vi "add scan field(SubVI).vi"(10 "字符串":string) -> (0 "布尔 3":bool, 2 "连接的字符串":string)   [LabVIEW 2019, in "Add Seq.lvlib"]
uses:
  Add Seq.lvlib
  SubVI.lvlib
panel:
  in  "Number of Step":i32=2
  in  "Step Delay(secs)":dbl
  in  "Increments(Oe)":dbl=10.0
  in  "cancel":bool
  in  "ok":bool
  in  "Approach":i32(ring)=1 items=["Linear", "NoOvershoot", "Oscillate", "Sweep"]
  in  "End Mode":i32(ring) items=["Persistent", "Driven"]
  in  "Rate(Oe/secs)":dbl=100.0 min=0.0 max=100.0
  in  "Final Field(Oe)":dbl min=-140000.0 max=140000.0
  in  "Initial Field(Oe)":dbl min=-140000.0 max=140000.0
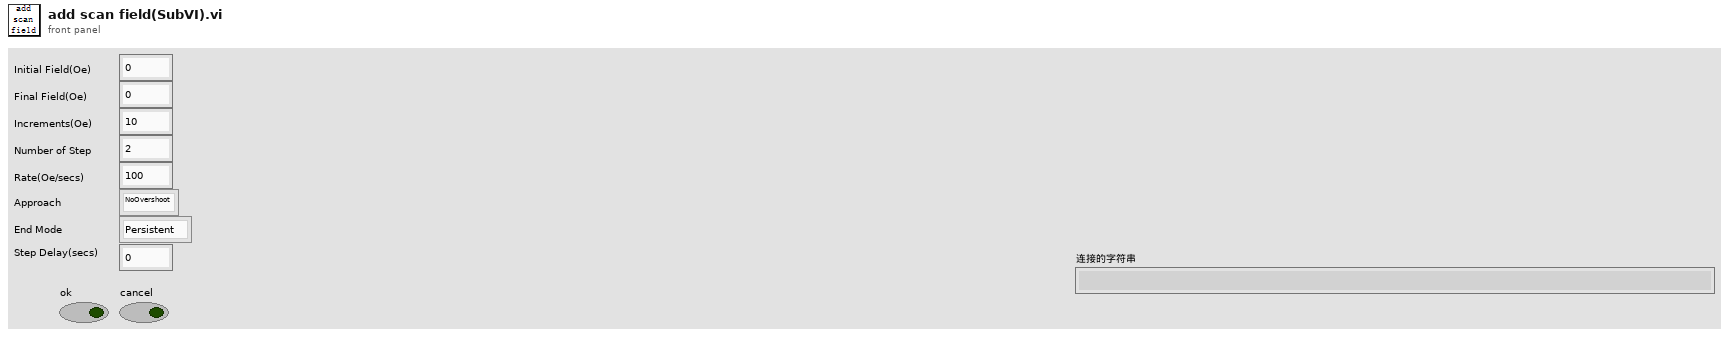
[diagram p1: front panel]
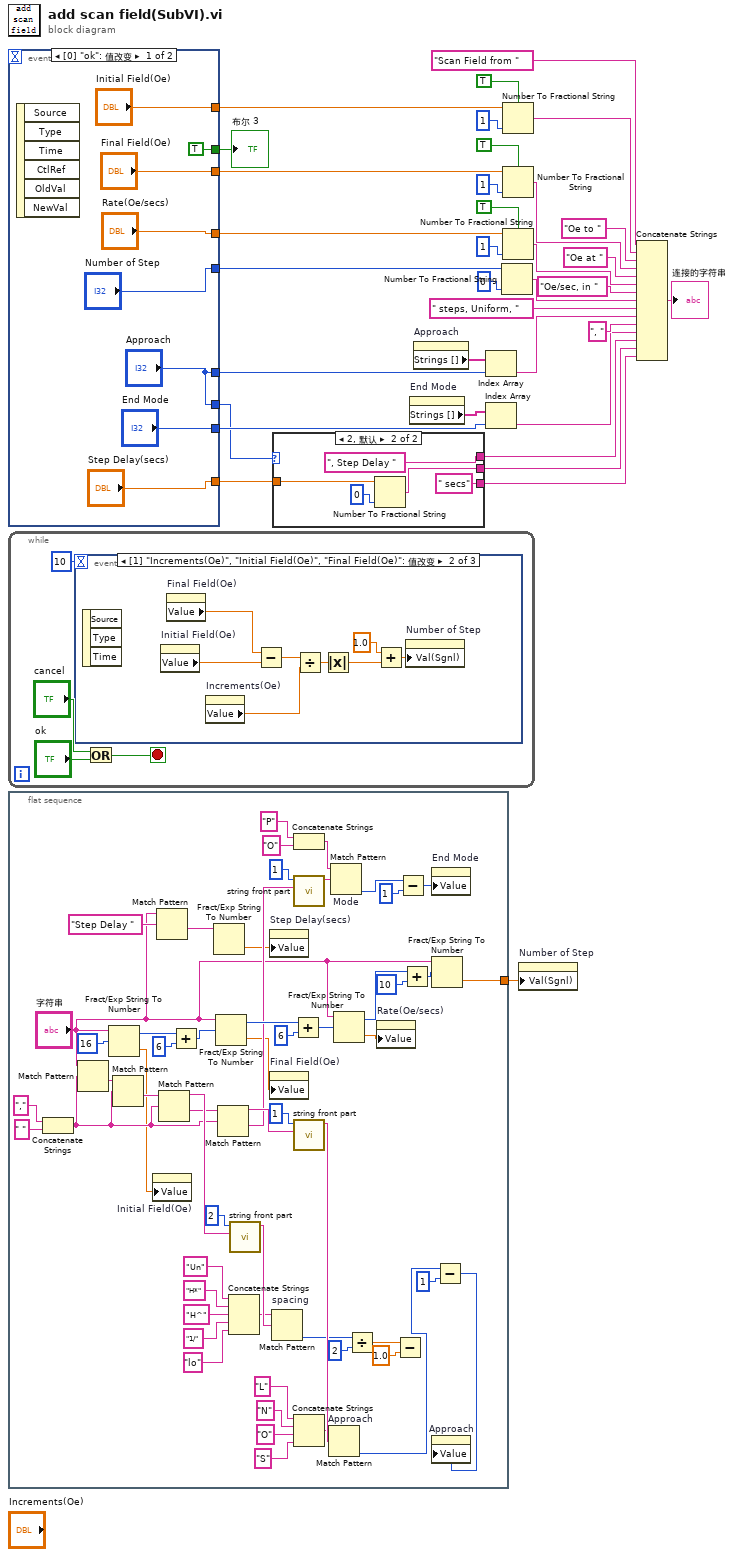
[diagram p0: block diagram]
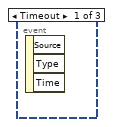
[diagram p2: hidden frame]
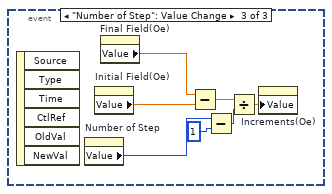
[diagram p3: hidden frame]
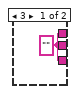
[diagram p4: hidden frame]
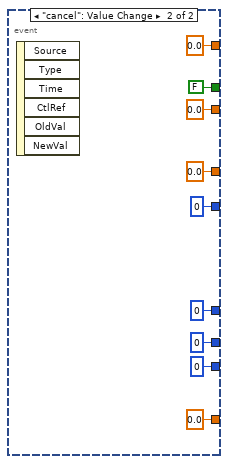
[diagram p5: hidden frame]
diagram:
  n1 = event shown="[0] \"ok\": 值改变" {
    selector: _ -> [_ _]
    dyn-events: _ -> [_ _]
    timeout: _ -> [_ _]
    tunnel: ["Final Field(Oe)" 0.0 ("Field 2")] -> w24
    tunnel: ["Rate(Oe/secs)" 0.0 ("Rate输入")] -> w21
    tunnel: ["Initial Field(Oe)" 0.0 ("Field")] -> w33
    tunnel: [TRUE FALSE] -> w35
    tunnel: ["Number of Step" 0 ("Number of Step")] -> w18
    tunnel: ["End Mode" 0 ("Mode输入")] -> w14
    tunnel: ["Approach" 0 ("Approach输入")] -> w11
    tunnel: ["Step Delay(secs)" 0.0 ("Step Delay(secs)")] -> w5
    tunnel: ["Approach" 0 ("Approach")] -> w3
    event "ok": Value Change {
      n2 = event-data() -> ()  [unwired: 1 in, 6 out]
    }
    event "cancel": Value Change {
      n3 = event-data() -> ()  [unwired: 1 in, 6 out]
    }
  }
  "布尔 3" <- w35
  n4 = while {
    stop <- w53 stop-if-true
    n5 = event shown="[1] \"Increments(Oe)\", \"Initial Field(Oe)\", \"Final Field(Oe)\": 值改变" {
      selector: _ -> [_ _ _]
      dyn-events: _ -> [_ _ _]
      timeout: 10 -> [_ _ _]
      event Timeout {
        n6 = event-data() -> ()  [unwired: 1 in, 3 out]
      }
      event "Increments(Oe)", "Initial Field(Oe)", "Final Field(Oe)": Value Change {
        n7 = event-data() -> ()  [unwired: 1 in, 3 out]
        n8 = property on="Initial Field(Oe)" class="DigNum (严格)"() -> ("Value"=w63:dbl)  [unwired: 2 in, 2 out]
        n9 = property on="Final Field(Oe)" class="DigNum (严格)"() -> ("Value"=w64:dbl)  [unwired: 2 in, 2 out]
        n10 = property on="Increments(Oe)" class="DigNum (严格)"() -> ("Value"=w61:dbl)  [unwired: 2 in, 2 out]
        n11 = Subtract(x=w64, y=w63) -> (x-y=w62:dbl)
        n12 = Divide(x=w62, y=w61) -> (x/y=w58:dbl)
        n13 = Absolute Value(x=w58) -> (abs(x)=w57:dbl)
        n14 = Add(x=1.0, y=w57) -> (x+y=w59:dbl)
        n15 = property on="Number of Step" class="DigNum (严格)"("Val(Sgnl)"=w59) -> ()  [unwired: 2 in, 2 out]
      }
      event "Number of Step": Value Change {
        n16 = event-data() -> ()  [unwired: 1 in, 6 out]
        n17 = property on="Number of Step" class="DigNum (严格)"() -> ("Value"=w68:i32)  [unwired: 2 in, 2 out]
        n18 = property on="Initial Field(Oe)" class="DigNum (严格)"() -> ("Value"=w70:dbl)  [unwired: 2 in, 2 out]
        n19 = property on="Final Field(Oe)" class="DigNum (严格)"() -> ("Value"=w71:dbl)  [unwired: 2 in, 2 out]
        n20 = Subtract(x=w71, y=w70) -> (x-y=w69:dbl)
        n21 = Subtract(x=w68, y=1) -> (x-y=w66:i32)
        n22 = Divide(x=w69, y=w66) -> (x/y=w65:dbl)
        n23 = property on="Increments(Oe)" class="DigNum (严格)"("Value"=w65) -> ()  [unwired: 2 in, 2 out]
      }
    }
    n24 = Or(x="cancel", y="ok") -> (x .or. y?=w53:bool)
  }
  n25 = flat-sequence {
    tunnel: [w75] -> w1
    frame #0 {
      n26 = Concatenate Strings("," ("字符串"), " " ("字符串")) -> (w87:string)
      n27 = Match Pattern(string="字符串", regular expression=w87) -> (after substring=w128:string)  [unwired: 1 in, 3 out]
      n28 = Fract/Exp String To Number(string="字符串", offset=16 ("偏移量")) -> (offset past number=w126:i32, number=w78:dbl)  [unwired: 2 in]
      n29 = Match Pattern(string=w128, regular expression=w87) -> (after substring=w103:string)  [unwired: 1 in, 3 out]
      n30 = property on="Initial Field(Oe)" class="DigNum (严格)"("Value"=w78) -> ()  [unwired: 2 in, 2 out]
      n31 = Match Pattern(string="字符串", regular expression="Step Delay ") -> (after substring=w83:string)  [unwired: 1 in, 3 out]
      n32 = Match Pattern(string=w103, regular expression=w87) -> (before substring=w102:string, after substring=w88:string)  [unwired: 1 in, 2 out]
      n33 = Add(x=w126, y=6) -> (x+y=w125:i32)
      n34 = Fract/Exp String To Number(string=w83) -> (number=w80:dbl)  [unwired: 3 in, 1 out]
      n35 = Fract/Exp String To Number(string="字符串", offset=w125) -> (offset past number=w108:i32, number=w77:dbl)  [unwired: 2 in]
      n36 = Match Pattern(string=w88, regular expression=w87) -> (before substring=w86:string, after substring=w85:string)  [unwired: 1 in, 2 out]
      n37 = Concatenate Strings("Un" ("字符串"), "H*" ("字符串"), "H^" ("字符串"), "1/" ("字符串"), "lo" ("字符串")) -> (w94:string)
      n38 = call "string front part.vi"("字符串"=w102, "偏移量(0)"=2) -> ("result string"=w100:string)  [unwired: 9 in]
      n39 = property on="Step Delay(secs)" class="DigNum (严格)"("Value"=w80) -> ()  [unwired: 2 in, 2 out]
      n40 = property on="Final Field(Oe)" class="DigNum (严格)"("Value"=w77) -> ()  [unwired: 2 in, 2 out]
      n41 = Match Pattern "spacing"(string=w94, regular expression=w100) -> (offset past match=w93:i32)  [unwired: 1 in, 3 out]
      n42 = Add(x=w108, y=6) -> (x+y=w106:i32)
      n43 = Concatenate Strings("P" ("字符串"), "O" ("字符串")) -> (w113:string)
      n44 = call "string front part.vi"("字符串"=w85, "偏移量(0)"=1) -> ("result string"=w116:string)  [unwired: 9 in]
      n45 = call "string front part.vi"("字符串"=w86, "偏移量(0)"=1) -> ("result string"=w122:string)  [unwired: 9 in]
      n46 = Concatenate Strings("L" ("字符串"), "N" ("字符串"), "O" ("字符串"), "S" ("字符串")) -> (w118:string)
      n47 = Match Pattern "Approach"(string=w118, regular expression=w122) -> (offset past match=w73:i32)  [unwired: 1 in, 3 out]
      n48 = Match Pattern "Mode"(string=w113, regular expression=w116) -> (offset past match=w112:i32)  [unwired: 1 in, 3 out]
      n49 = Fract/Exp String To Number(string="字符串", offset=w106) -> (offset past number=w89:i32, number=w76:dbl)  [unwired: 2 in]
      n50 = Divide(x=w93, y=2) -> (x/y=w91:dbl)
      n51 = property on="Rate(Oe/secs)" class="DigNum (严格)"("Value"=w76) -> ()  [unwired: 2 in, 2 out]
      n52 = Subtract(x=w91, y=1.0) -> ()  [unwired: 1 out]
      n53 = Subtract(x=w112, y=1) -> (x-y=w79:i32)
      n54 = Add(x=w89, y=10) -> (x+y=w104:i32)
      n55 = property on="End Mode" class="Ring (严格)"("Value"=w79) -> ()  [unwired: 2 in, 2 out]
      n56 = Fract/Exp String To Number(string="字符串", offset=w104) -> (number=w75:dbl)  [unwired: 2 in, 1 out]
      n57 = Subtract(x=w73, y=1) -> (x-y=w72:i32)
      n58 = property on="Approach" class="Ring (严格)"("Value"=w72) -> ()  [unwired: 2 in, 2 out]
    }
  }
  n59 = case shown="2, 默认" w3 {
    tunnel: [w129 ", Step Delay " ("字符串")] -> w7
    tunnel: [w129 " secs" ("字符串")] -> w6
    tunnel: w5 -> [_ w132]
    tunnel: [w129 w131] -> w4
    frame 3 {
      w129 = ""
    }
    frame 2, Default {
      n60 = Number To Fractional String(number=w132, precision (6)=i16 0 ("精度(6)")) -> (F-format string=w131:string)  [unwired: 2 in]
    }
  }
  n61 = property on="End Mode" class="Ring (严格)"() -> ("Strings []"=w15:string[])  [unwired: 2 in, 2 out]
  n62 = property on="Approach" class="Ring (严格)"() -> ("Strings []"=w12:string[])  [unwired: 2 in, 2 out]
  n63 = Index Array(array=w12, index=w11) -> (element=w8:string)
  n64 = Index Array(array=w15, index=w14) -> (element=w9:string)
  n65 = Number To Fractional String(number=w18, precision (6)=i16 0 ("精度(6)")) -> (F-format string=w17:string)  [unwired: 2 in]
  n66 = Number To Fractional String(use system decimal point (T)=TRUE ("使用系统小数点(T)"), number=w33, precision (6)=i16 1 ("精度(6)")) -> (F-format string=w31:string)  [unwired: 1 in]
  n67 = Number To Fractional String(use system decimal point (T)=TRUE ("使用系统小数点(T)"), number=w24, precision (6)=i16 1 ("精度(6)")) -> (F-format string=w26:string)  [unwired: 1 in]
  n68 = Number To Fractional String(use system decimal point (T)=TRUE ("使用系统小数点(T)"), number=w21, precision (6)=i16 1 ("精度(6)")) -> (F-format string=w20:string)  [unwired: 1 in]
  n69 = property on="Number of Step" class="DigNum (严格)"("Val(Sgnl)"=w1) -> ()  [unwired: 2 in, 2 out]
  n70 = Concatenate Strings("Scan Field from " ("字符串"), w31, "Oe to " ("字符串"), w26, "Oe at " ("字符串"), w20, "Oe/sec, in " ("字符串"), w17, " steps, Uniform, " ("字符串"), w8, ", " ("字符串"), w9, w7, w4, w6) -> (→"连接的字符串":string)
